vi "Overlay Result.vi"(6 "Processing Time":dbl, 8 "error in (no error)":errorcluster, 9 "Results":T1, 10 "Treatment":T2, 11 "Images":T3) -> (0 "error out":errorcluster, 1 "Results Out":T1, 2 "Treatment Out":T2, 3 "Images":T3)   [LabVIEW 2015]
uses:
  controls/Results.ctl
  <vilib>/vision/Image Controls.llb/IMAQ Image.ctl
  controls/Treatment Parameters.ctl
  controls/Images.ctl
panel:
  out "Overlaid Image":T4
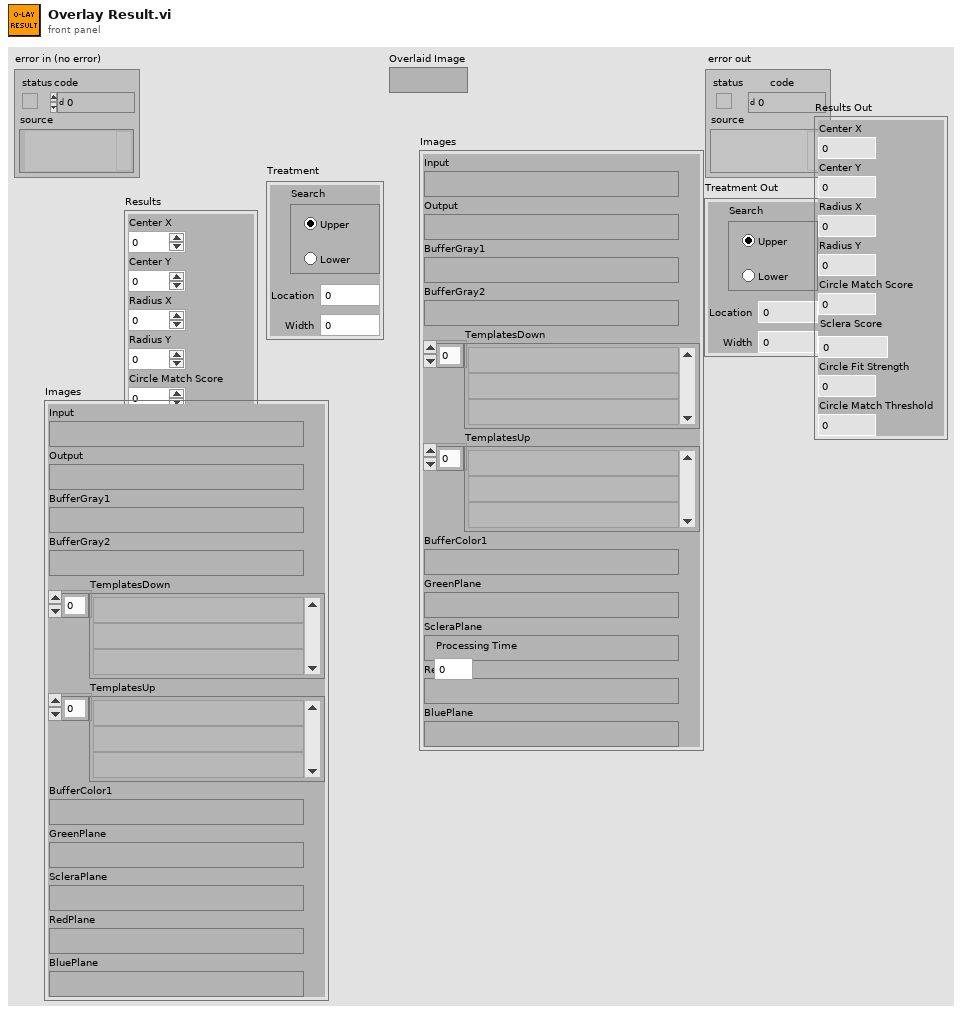
[diagram p1: front panel]
types:
  T1 = typedef "Results.ctl" = cluster{"Center X":i32, "Center Y":i32, "Radius X":i32, "Radius Y":i32, "Circle Match Score":i32, "Sclera Score":dbl, "Circle Fit Strength":i32, "Circle Match Threshold":i32}
  T2 = typedef "Treatment Parameters.ctl" = cluster{"Location":dbl, "Width":dbl, "Search":enum32{"Upper", "Lower"}}
  T3 = typedef "Images.ctl" = cluster{"Input":T4, "Output":T4, "BufferGray1":T4, "BufferGray2":T4, "TemplatesDown":T4[], "TemplatesUp":T4[], "BufferColor1":T4, "GreenPlane":T4, "ScleraPlane":T4, "RedPlane":T4, "BluePlane":T4}
  T4 = typedef "IMAQ Image.ctl" = refnum<image>
  T5 = cluster{"Desired Font (Application)":enum16{"User-specified Font", "Application Font", "System Font", "Dialog Font"}, "[User-specified Font]":cluster{"Font Name":string, "Size":i16, "Strikeout?":bool, "Italic?":bool, "Underline?":bool, "Outline?":bool, "Shadow?":bool, "Bold?":bool, "Rotation Angle":dbl}, "Horizontal Alignment":i16, "Vertical Alignment":i16}
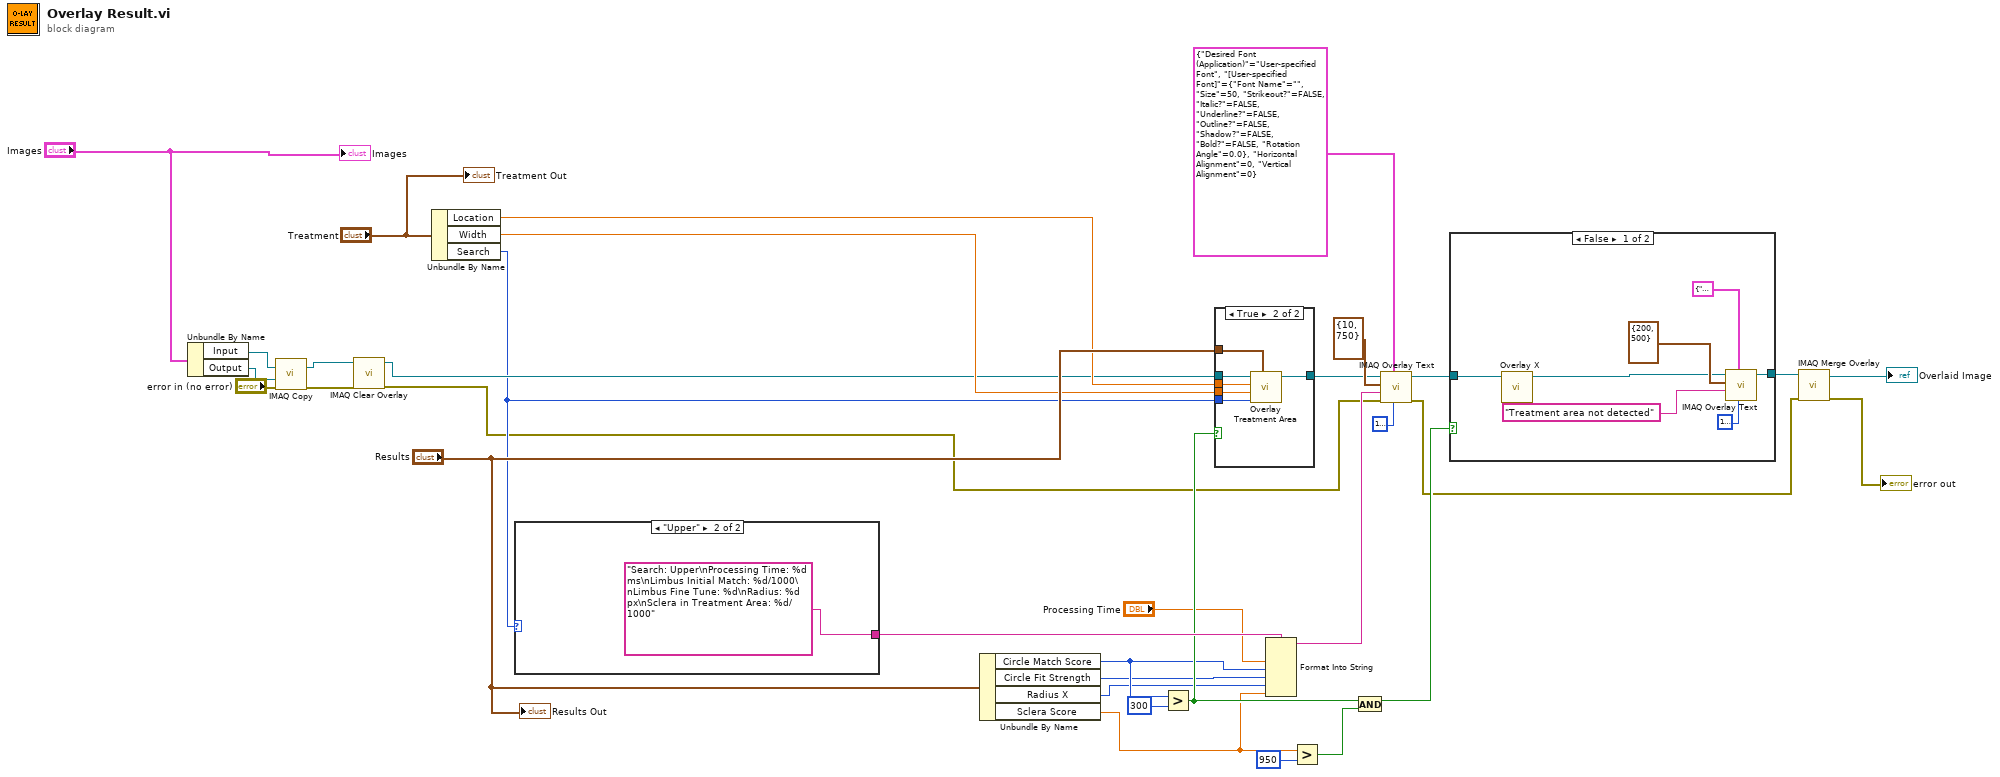
[diagram p0: block diagram]
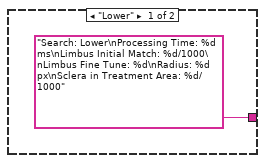
[diagram p4: hidden frame]
diagram:
  n1 = Unbundle By Name("Images") -> ("Input"=w11:T4, "Output"=w10:T4)
  n2 = call "IMAQ Copy"("error in (no error)"="error in (no error)", "Image Dst"=w10, "Image Src"=w11) -> ("error out"=w16:errorcluster, "Image Dst Out"=w17:T4)  [unwired: 3 in]
  n3 = call "IMAQ Clear Overlay"("error in (no error)"=w16, "Image"=w17) -> ("error out"=w8:errorcluster, "Image Out"=w15:T4)  [unwired: 8 in]
  n4 = Unbundle By Name("Treatment") -> ("Location"=w30:dbl, "Width"=w29:dbl, "Search"=w14:enum32{"Upper", "Lower"})
  n5 = case shown="\"Upper\"" w14 {
    tunnel: ["Search: Lower\nProcessing Time: %d ms\nLimbus Initial Match: %d/1000\nLimbus Fine Tune: %d\nRadius: %d px\nSclera in Treatment Area: %d/1000" ("String") "Search: Upper\nProcessing Time: %d ms\nLimbus Initial Match: %d/1000\nLimbus Fine Tune: %d\nRadius: %d px\nSclera in Treatment Area: %d/1000" ("String")] -> w32
    frame "Lower" {
    }
    frame "Upper" {
    }
  }
  n6 = Unbundle By Name("Results") -> ("Circle Match Score"=w4:i32, "Circle Fit Strength"=w3:i32, "Radius X"=w2:i32, "Sclera Score"=w1:dbl)
  n7 = Greater?(x=w4, y=300) -> (0:w13:bool)
  n8 = case shown="True" w13 {
    tunnel: "Results" -> [_ w43]
    tunnel: w30 -> [_ w42]
    tunnel: w29 -> [_ w41]
    tunnel: [w37 w40] -> w24
    tunnel: w15 -> [w37 w39]
    tunnel: w14 -> [_ w38]
    frame False {
    }
    frame True {
      n9 = call "Overlay Treatment Area.vi"("Results"=w43, "Search"=w38, "Width"=w41, "Location"=w42, "Refnum in"=w39) -> ("Refnum out"=w40:T4)  [unwired: 6 in]
    }
  }
  n10 = Format Into String(format string=w32, "Processing Time", w4, w3, w2, w1) -> (resulting string=w28:string)  [unwired: 2 in, 1 out]
  n11 = Greater?(x=w1, y=950) -> (0:w18:bool)
  n12 = And(x=w13, y=w18) -> (x .and. y?=w19:bool)
  n13 = call "IMAQ Overlay Text"("Text Color (black)"=u32 16777222 ("Color"), "Font, Size & Style"=T5 {"Desired Font (Application)"=enum."User-specified Font", "[User-specified Font]"={"Font Name"="", "Size"=50, "Strikeout?"=FALSE, "Italic?"=FALSE, "Underline?"=FALSE, "Outline?"=FALSE, "Shadow?"=FALSE, "Bold?"=FALSE, "Rotation Angle"=0.0}, "Horizontal Alignment"=0, "Vertical Alignment"=0}, "error in (no error)"=w8, "String"=w28, "Origin"=cluster{"X":i32, "Y":i32} {"X"=10, "Y"=750}, "Image"=w24) -> ("error out"=w7:errorcluster, "Image Out"=w22:T4)  [unwired: 4 in]
  n14 = case shown="False" w19 {
    tunnel: [w45 w51] -> w23
    tunnel: w22 -> [w44 w51]
    frame False {
      n15 = call "Overlay X.vi"("Refnum in"=w44) -> ("Refnum out"=w47:T4)  [unwired: 10 in]
      n16 = call "IMAQ Overlay Text"("Text Color (black)"=u32 16777222 ("Color"), "Font, Size & Style"=T5 {"Desired Font (Application)"=enum."User-specified Font", "[User-specified Font]"={"Font Name"="", "Size"=70, "Strikeout?"=FALSE, "Italic?"=FALSE, "Underline?"=FALSE, "Outline?"=FALSE, "Shadow?"=FALSE, "Bold?"=FALSE, "Rotation Angle"=0.0}, "Horizontal Alignment"=0, "Vertical Alignment"=0}, "String"="Treatment area not detected", "Origin"=cluster{"X":i32, "Y":i32} {"X"=200, "Y"=500}, "Image"=w47) -> ("Image Out"=w45:T4)  [unwired: 5 in, 1 out]
    }
    frame True {
    }
  }
  n17 = call "IMAQ Merge Overlay"("error in (no error)"=w7, "Image Src"=w23) -> ("error out"=→"error out":errorcluster, "Image Dst Out"=→"Overlaid Image":T4)  [unwired: 8 in]
  "Images" <- "Images"
  "Treatment Out" <- "Treatment"
  "Results Out" <- "Results"
